vi "PadAreaStringsVar.vi"() -> ()   [LabVIEW 2012]
uses:
  Controls/PadAreaItemStrings.ctl
panel:
  in  "Strings []":T1=["A", "B", "C", "D", "L", "R", "T", "G"]
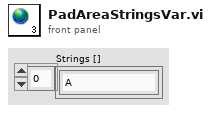
[diagram p1: front panel]
types:
  T1 = typedef "PadAreaItemStrings.ctl" = string[]
diagram:
